vi "Mono_CheckStatud.vi"(8 "error in (no error) 2":errorcluster, 11 "CmdLib In":refnum<k24>) -> (0 "error out 2":errorcluster, 1 "getWavelength":dbl, 3 "CmdLib Out":refnum<k24>)   [LabVIEW 2023]
uses:
  E:/Old PC/desktop/Sensitive EQE Stuff/S-EQE (YJ)/Mono vi (YJ)/Cornerstone.dll
  Cornerstone.dll
panel:
  out "getResponse":string
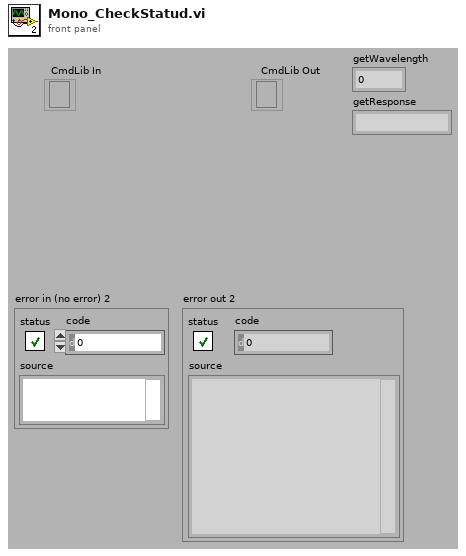
[diagram p1: front panel]
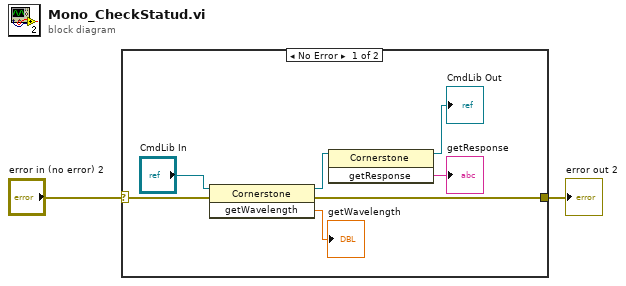
[diagram p0: block diagram]
diagram:
  n1 = case shown="No Error" "error in (no error) 2" {
    selector: "error in (no error) 2" -> [w9 w10]
    tunnel: [w4 w10] -> w1
    frame No Error {
      n2 = invoke class="Cornerstone" method="getWavelength"(reference="CmdLib In", error in=w9) -> (reference out=w6:refnum<k24>, error out=w4:errorcluster, "getWavelength"=→"getWavelength":dbl)  [unwired: 1 in]
      n3 = invoke class="Cornerstone" method="getResponse"(reference=w6) -> (reference out=→"CmdLib Out":refnum<k24>, "getResponse"=→"getResponse":string)  [unwired: 2 in, 1 out]
    }
    frame Error {
    }
  }
  "error out 2" <- w1
